vi "Column wash timer.vi"(5 "УЗ7":dbl format="%#_13g", 7 "СЧ1":dbl) -> (4 "Насос 3":bool=TRUE, 6 "КР1":dbl format="%#_13g", 8 "Насос 8":bool=TRUE, 10 "Error output":bool, 15 "Status":bool)   [LabVIEW 2019]
panel:
  # "Выход"
  # "Вход"
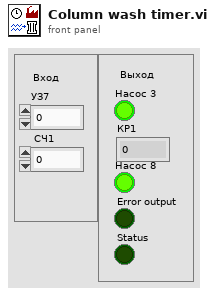
[diagram p1: front panel]
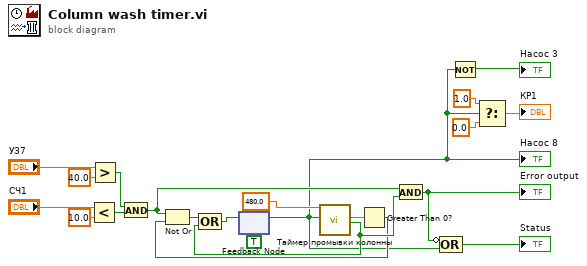
[diagram p0: block diagram]
diagram:
  n1 = Less?(x="СЧ1", y=10.0) -> (x < y?=w9:bool)
  n2 = Greater?(x="УЗ7", y=40.0) -> (0:w7:bool)
  n3 = And(x=w7, y=w9) -> (x .and. y?=w8:bool)
  n4 = feedback #1(TRUE) -> (w2:bool)
  "Насос 8" <- w2
  n5 = call "Таймер промывки колонны"("Time Target (s)"=480.0, "Reset"=w2) -> ("Elapsed Time (s)"=w16:dbl, "Time has Elapsed"=w20:bool)  [unwired: 10 in, 6 out]
  n6 = Greater Than 0?(x=w16) -> (x > 0?=w18:bool)
  n7 = Not Or(1:w18, 2:w8) -> (0:w19:bool)
  n8 = Compound Arithmetic op=OR(w19, w20) -> (w21:bool)
  n9 = feedback-in #1(w21) -> ()
  n10 = And(x=w8, y=w20) -> (x .and. y?=w6:bool)
  "Error output" <- w6
  n11 = Compound Arithmetic op=OR(invert w6, w2) -> (→"Status":bool)
  n12 = Not(x=w2) -> (.not. x?=→"Насос 3":bool)
  n13 = Select(t=1.0, s=w2, f=0.0) -> (s? t:f=→"КР1":dbl)
